vi "Initialize waveplate.vi"(8 "error in (no error)":errorcluster, 10 "Axis in":i32, 11 "VISA Handle in":refnum<visa-resource-name>) -> (0 "error out":errorcluster, 2 "WP Error":bool=TRUE, 3 "VISA Refnum out":refnum<visa-resource-name>)   [LabVIEW 2013]
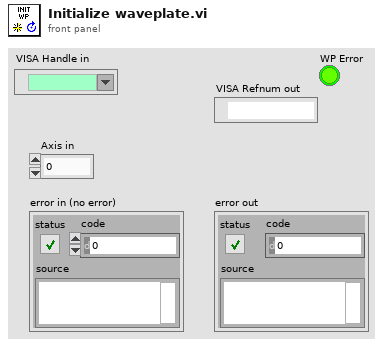
[diagram p1: front panel]
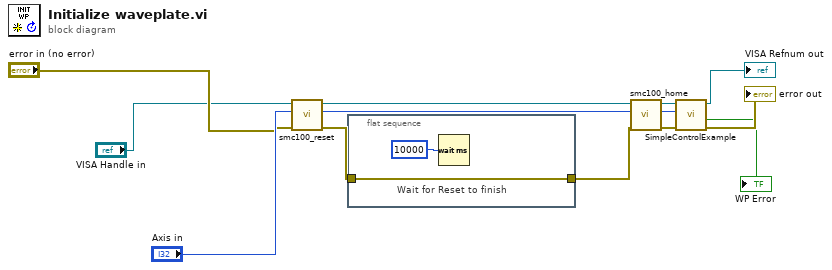
[diagram p0: block diagram]
diagram:
  n1 = call "smc100_reset.vi"("error in"="error in (no error)", "Axis in"="Axis in", "VISA Handle in"="VISA Handle in") -> ("error out"=w8:errorcluster, "Axis out"=w7:i32, "VISA Handle out"=w13:refnum<visa-resource-name>)  [unwired: 3 in, 1 out]
  n2 = flat-sequence {
    tunnel: [w14] -> w9
    tunnel: w8 -> [w14]
    frame #0 {
      # "Wait for Reset to finish"
      n3 = Wait (ms)(milliseconds to wait=u32 10000) -> ()  [unwired: 1 out]
    }
  }
  n4 = call "smc100_home.vi"("error in"=w9, "Axis in"=w7, "VISA Handle in"=w13) -> ("error out"=w5:errorcluster, "Axis out"=w6:i32, "VISA Handle out"=w4:refnum<visa-resource-name>)  [unwired: 3 in, 1 out]
  n5 = call "SimpleControlExample.vi"("error in"=w5, "Axis in"=w6, "VISA Handle in"=w4) -> ("error out"=→"error out":errorcluster, "WP Error"=→"WP Error":bool, "VISA Handle out"=→"VISA Refnum out":refnum<visa-resource-name>)  [unwired: 2 in, 2 out]
